vi "Global Stop.vi"(7 "Operation":T1=enum."Init", 8 "error in (no error)":errorcluster) -> (0 "error out":errorcluster, 3 "Stop?":bool)   [LabVIEW 2011]
uses:
  Controls/Global Stop - Operations.ctl
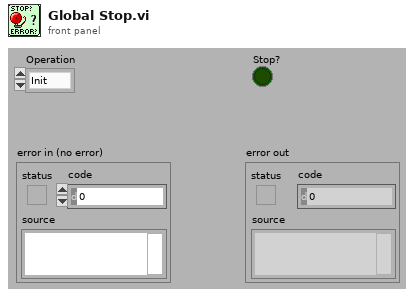
[diagram p1: front panel]
types:
  T1 = typedef "Global Stop - Operations.ctl" = enum16{"Stop", "Status", "Init"}
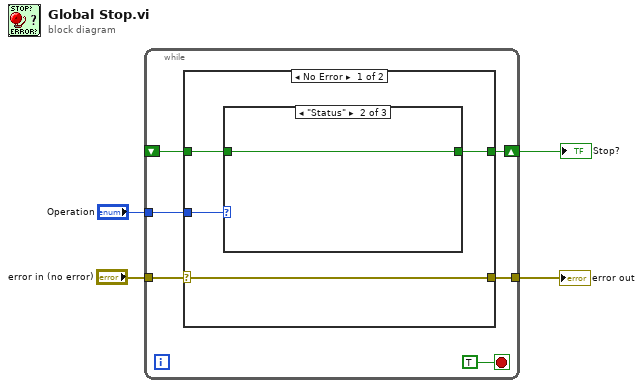
[diagram p0: block diagram]
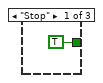
[diagram p2: hidden frame]
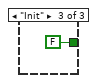
[diagram p3: hidden frame]
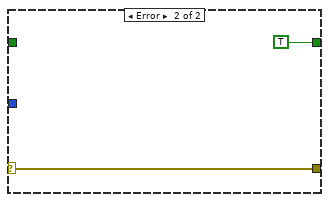
[diagram p4: hidden frame]
diagram:
  n1 = while {
    tunnel: "Operation" -> [w6]
    tunnel: "error in (no error)" -> [w9]
    tunnel: [w8] -> w2
    shift-right: [w7] -> w1
    shift-left: _ -> [w5]
    stop <- TRUE stop-if-true
    n2 = case shown="No Error" w9 {
      selector: w9 -> [w14 w18]
      tunnel: [w14 w18] -> w8
      tunnel: [w11 TRUE] -> w7
      tunnel: w6 -> [w13 _]
      tunnel: w5 -> [w12 _]
      frame No Error {
        n3 = case shown="\"Status\"" w13 {
          tunnel: w12 -> [_ w16 _]
          tunnel: [TRUE w16 FALSE] -> w11
          frame "Stop" {
          }
          frame "Status" {
          }
          frame "Init" {
          }
        }
      }
      frame Error {
      }
    }
  }
  "error out" <- w2
  "Stop?" <- w1
